vi "Deconstruct.vi"(0 "User Configuration Manager in":refnum<class "User Configuration Manager.lvclass">, 11 "error in (no error)":errorcluster) -> (15 "error out":errorcluster)   [LabVIEW 2020, in "User Configuration Manager.lvlib" / "User Configuration Manager.lvclass"]
uses:
  <vilib>/gpm_packages/@cs/user-manager/Source/User Configuration Manager/User Configuration Manager.lvclass
  <vilib>/gpm_packages/@cs/user-manager/Source/User Configuration Manager/User Configuration Manager.lvclass/User Configuration Manager.ctl
  <vilib>/gpm_packages/@cs/linked-list/Source/Linked List/Linked List Ref/Linked List Ref.lvclass
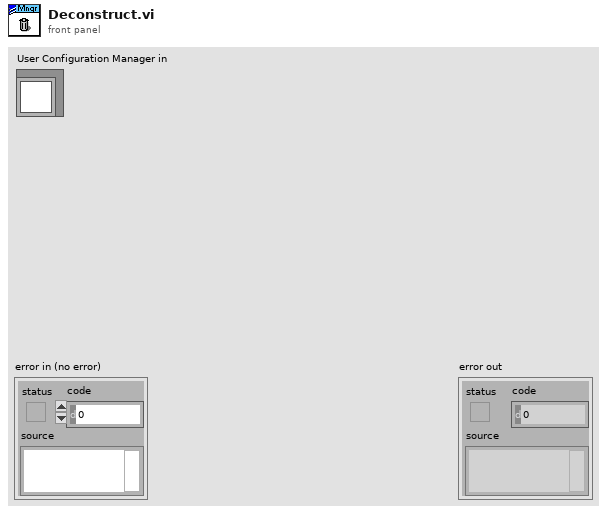
[diagram p1: front panel]
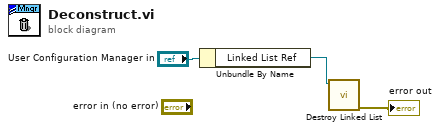
[diagram p0: block diagram]
diagram:
  n1 = Unbundle By Name("User Configuration Manager in") -> ("Linked List Ref"=w1:refnum<data-value>)
  n2 = call <vilib>:"Destroy Linked List.vi"("Linked List Ref"=w1) -> ("error out"=→"error out":errorcluster)  [unwired: 10 in]
